vi "Rotate To Target.vi"() -> (0 "On Target":bool)   [LabVIEW 2015]
uses:
  <vilib>/Rock Robotics/WPI/SafetyOutput/WPI_SafetyOutputConfigMenu.ctl
  Robot Global Data.vi
  <vilib>/Rock Robotics/WPI/Utilities/WPI_GetSetVariantRefNum.vi
  <vilib>/Rock Robotics/WPI/RobotDrive/WPI_RobotDriveArcadeDrive_Standard(NoSaturation).vi
  <vilib>/Rock Robotics/Network Tables/NT Write Numeric Array.vi
panel:
  in  "Y Tolerance (px)":i16=10
  in  "X Tolerance (px)":i16=3
  in  "Target Y":i16=180
  in  "Target X":i16=155
  out "Image":T1(plugin-control)
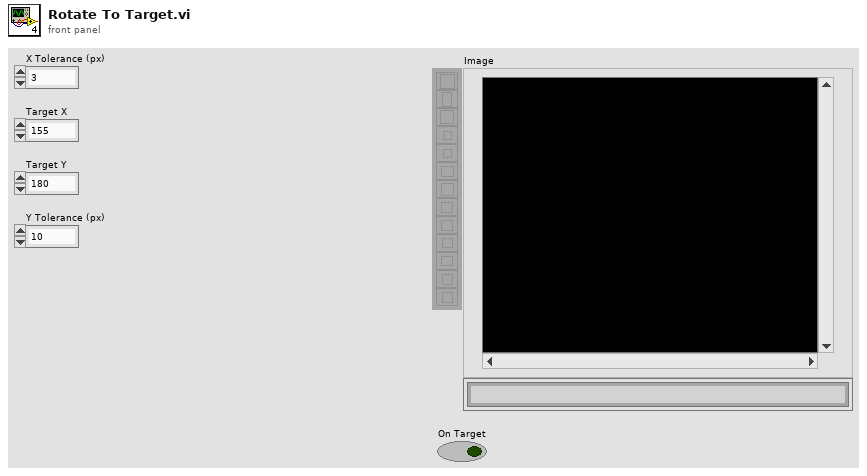
[diagram p1: front panel]
types:
  T1 = typedef "IMAQ Image.ctl" = refnum<image>
  T2 = typedef "WPI_SafetyOutputConfigMenu.ctl" = enum16{"Enable", "Disable"}
  T3 = typedef "Image Type" = u32
  T4 = typedef "WPI_RobotDriveDevRef.ctl" = cluster{"DevStatus":errorcluster, "Motors[]":T5[], "Square Inputs":bool, "Max Output":dbl}
  T5 = typedef "WPI_MotorControlDeviceRef.ctl" = cluster{"DeviceStatus":errorcluster, "Type":T6, "PWM":cluster{"PWM Channel":T7, "DeadBand":T8}, "CAN":cluster{"Device Number":u8, "Control Mode":T9, "Semaphore":T10, "Max Vout":dbl, "TalonSRX Control Mode":T11}, "Invert":bool}
  T6 = typedef "WPI_MotorControlType.ctl" = enum16{"PWM", "CAN", "CANTalonSRX"}
  T7 = typedef "FPGA_DIOPWMChannel.ctl" = enum8{"PWM 0", "PWM 1", "PWM 2", "PWM 3", "PWM 4", "PWM 5", "PWM 6", "PWM 7", "PWM 8", "PWM 9", "PWM MXP 0", "PWM MXP 1", "PWM MXP 2", "PWM MXP 3", "PWM MXP 4", "PWM MXP 5", "PWM MXP 6", "PWM MXP 7", "PWM MXP 8", "PWM MXP 9", "Invalid"}
  T8 = typedef "WPI_PWMDeadband.ctl" = cluster{"Name":string, "maxPositivePwm":i32, "minPositivePwm":i32, "centerPwm":i32, "maxNegativePwm":i32, "minNegativePwm":i32, "angularRange":u16}
  T9 = typedef "WPI_CANJaguar_ControlMode.ctl" = enum8{"Percent VBus", "Current", "Speed", "Position", "Voltage"}
  T10 = typedef "Semaphore RefNum" = refnum<k1>
  T11 = typedef "WPI_CANTalonSRX_APIControlMode.ctl" = enum8{"Percent VBus", "Speed", "Position", "Slave", "Unchanged / Invalid", "Voltage Compensation", "Current", "Motion Profile"}
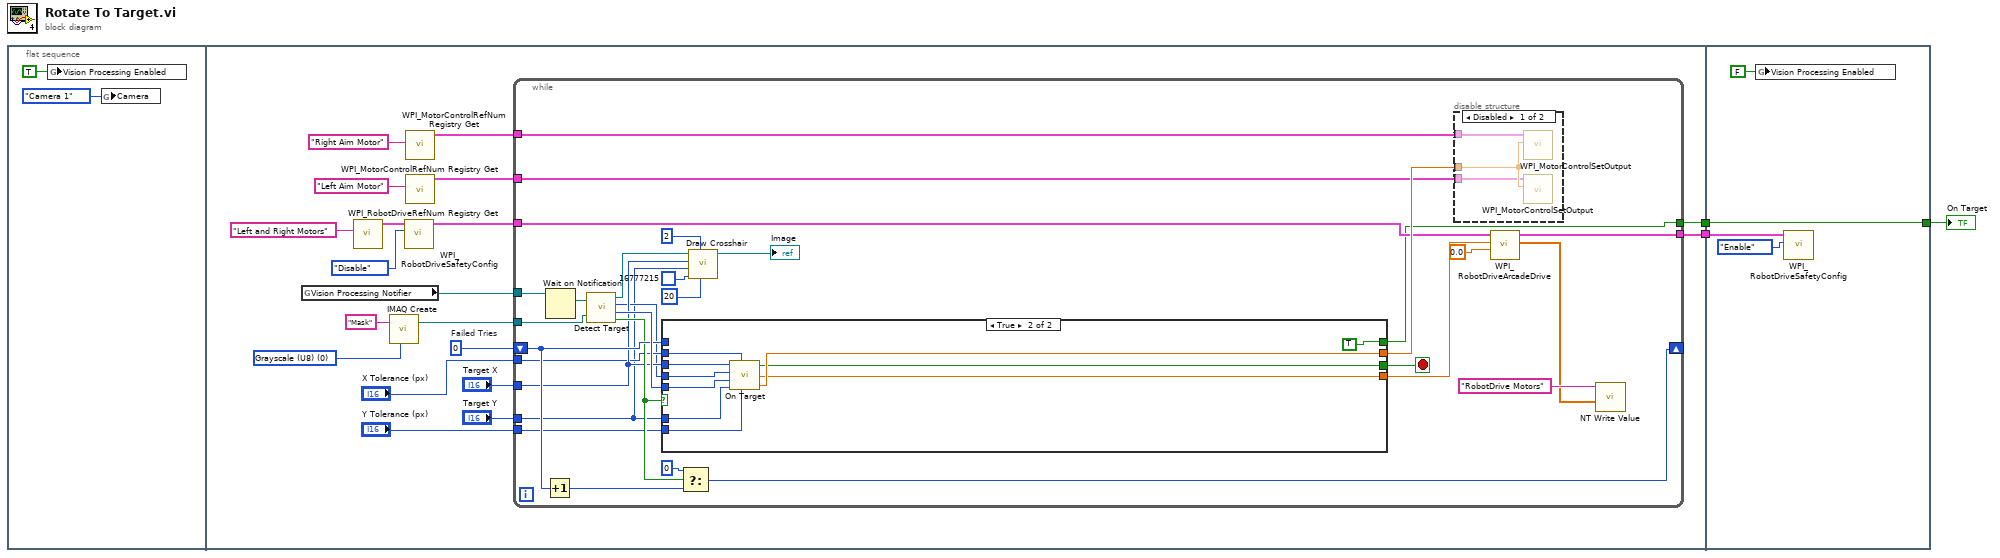
[diagram p0: block diagram]
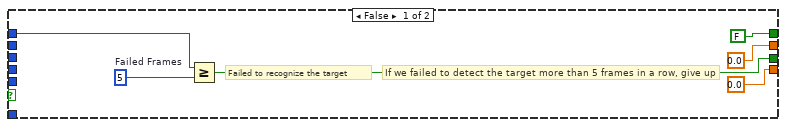
[diagram p3: hidden frame]
diagram:
  n1 = flat-sequence {
    tunnel: [w7] -> w3
    tunnel: [w6] -> w1
    tunnel: w3 -> [w77]
    tunnel: [w77] -> w2
    tunnel: w1 -> [w76]
    frame #0 {
      n2 = global write "Robot Global Data.vi" "Vision Processing Enabled"(TRUE ("Vision Processing Enabled")) -> ()
      n3 = global write "Robot Global Data.vi" "Camera"(enum16{"Camera 1", "Camera 2"}."Camera 1" ("Camera")) -> ()
    }
    frame #1 {
      w20 = 0  # Failed Tries
      w17 = T3 0 items=["Grayscale (U8)", "Grayscale (I16)", "Grayscale (SGL)", "Complex (CSG)", "RGB (U32)", "HSL (U32)", "RGB (U64)", "Grayscale (U16)"] ("Image Type")
      n4 = global read "Robot Global Data.vi" "Vision Processing Notifier"() -> (w16:refnum<notifier>)
      n5 = call <vilib>:"WPI_RobotDriveRefNum Registry Get.vi"("refnum name"="Left and Right Motors") -> ("RobotDriveDevRef"=w9:T4)  [unwired: 1 in, 9 out]
      n6 = call "IMAQ Create"("Image Name"="Mask", "Image Type"=w17) -> ("New Image"=w19:T1)  [unwired: 2 in, 2 out]
      n7 = call <vilib>:"WPI_RobotDriveSafetyConfig.vi"("mode"=WPI_SafetyOutputConfigMenu."Disable", "RobotDriveDevRef"=w9) -> ("RobotDriveDevRef"=w8:T4)  [unwired: 8 in, 1 out]
      n8 = call <vilib>:"WPI_MotorControlRefNum Registry Get.vi"("refnum name"="Right Aim Motor") -> ("MotorControlDevRef"=w12:T5)  [unwired: 9 in, 1 out]
      n9 = call <vilib>:"WPI_MotorControlRefNum Registry Get.vi"("refnum name"="Left Aim Motor") -> ("MotorControlDevRef"=w13:T5)  [unwired: 9 in, 1 out]
      n10 = while {
        tunnel: w16 -> [w54]
        tunnel: w19 -> [w52]
        shift-right: [w50] -> _
        shift-left: w20 -> [w35]
        tunnel: "Target Y" -> [w28]
        tunnel: "Target X" -> [w32]
        tunnel: w8 -> [w37]
        tunnel: [w33] -> w7
        tunnel: "X Tolerance (px)" -> [w31]
        tunnel: "Y Tolerance (px)" -> [w29]
        tunnel: w13 -> [w27]
        tunnel: w12 -> [w26]
        tunnel: [w25] -> w6
        stop <- w36 stop-if-true
        n11 = Increment(x=w35) -> (x+1=w48:i32)
        n12 = Wait on Notification(notifier=w54) -> (notification=w53:T1)  [unwired: 2 in, 4 out]
        n13 = call "Detect Target.vi"("Image"=w53, "Image Mask"=w52) -> ("Original Image"=w43:T1, "X"=w30:i16, "Y"=w51:i16, "Found Target"=w34:bool)
        n14 = case shown="True" w34 {
          tunnel: w51 -> [_ w66]
          tunnel: [0.0 w73] -> w47
          tunnel: w28 -> [_ w64]
          tunnel: [0.0 w68] -> w40
          tunnel: [w59 w69] -> w36
          tunnel: w35 -> [w60 _]
          tunnel: [FALSE TRUE] -> w33
          tunnel: w32 -> [_ w65]
          tunnel: w31 -> [_ w71]
          tunnel: w30 -> [_ w67]
          tunnel: w29 -> [_ w70]
          frame False {
            w61 = 5  # Failed Frames
            # "If we failed to detect the target more than 5 frames in a row, give up"
            # "Failed to recognize the target"
            n15 = Greater Or Equal?(x=w60, y=w61) -> (x >= y?=w59:bool)
          }
          frame True {
            n16 = call "On Target.vi"("Target X"=w65, "X Tolerance"=w71, "X"=w67, "Y"=w66, "Y Tolerance"=w70, "Target Y"=w64) -> ("Horizontal In Range"=w69:bool, "Turn Speed"=w68:dbl, "Arm Lift Speed"=w73:dbl)
          }
        }
        n17 = Select(t=0, s=w34, f=w48) -> (s? t:f=w50:i32)
        n18 = call "Draw Crosshair.vi"("Length"=20, "Thickness"=2, "Color"=u32 16777215, "Y"=w28, "X"=w32, "Image in"=w43) -> ("Image out"=→"Image":T1)  [unwired: 5 in]
        n19 = disable-structure shown="Disabled" {
          disable-tunnel: w47 -> [w57 _]
          disable-tunnel: w27 -> [w56 _]
          disable-tunnel: w26 -> [w55 _]
          frame Disabled {
            n20 = call <vilib>:"WPI_MotorControlSetOutput.vi"("Output"=w57, "MotorControlDevRef"=w55) -> ()  [unwired: 7 in, 3 out]
            n21 = call <vilib>:"WPI_MotorControlSetOutput.vi"("Output"=w57, "MotorControlDevRef"=w56) -> ()  [unwired: 7 in, 3 out]
          }
          frame Enabled {
          }
        }
        n22 = call-poly <vilib>:"WPI_RobotDriveArcadeDrive.vi"("Y axis value"=0.0, "X axis value"=w40, "RobotDriveDevRef"=w37) -> ("Motor Values"=w38:dbl[], "RobotDriveDevRef"=w25:T4)  [unwired: 1 in, 6 out]
        n23 = call-poly <vilib>:"NT Write Value.vi"("Numeric Array"=w38, "Name"="RobotDrive Motors") -> ()  [unwired: 9 in, 1 out]
      }
    }
    frame #2 {
      n24 = global write "Robot Global Data.vi" "Vision Processing Enabled"(FALSE ("Vision Processing Enabled")) -> ()
      n25 = call <vilib>:"WPI_RobotDriveSafetyConfig.vi"("mode"=WPI_SafetyOutputConfigMenu."Enable", "RobotDriveDevRef"=w76) -> ()  [unwired: 8 in, 2 out]
    }
  }
  "On Target" <- w2
